vi "Obtain Future.vi"(8 "error in (no error)":errorcluster, 9 "create if not found? (T)":bool=TRUE, 10 "name (unnamed)":string, 11 "Future in":refnum<class "Future.lvclass">) -> (0 "error out":errorcluster, 1 "created new?":bool, 3 "Future out":refnum<class "Future.lvclass">)   [LabVIEW 2017, in "Promise Future.lvlib" / "Future.lvclass"]
uses:
  Future.lvclass
  Future.lvclass/Future.ctl
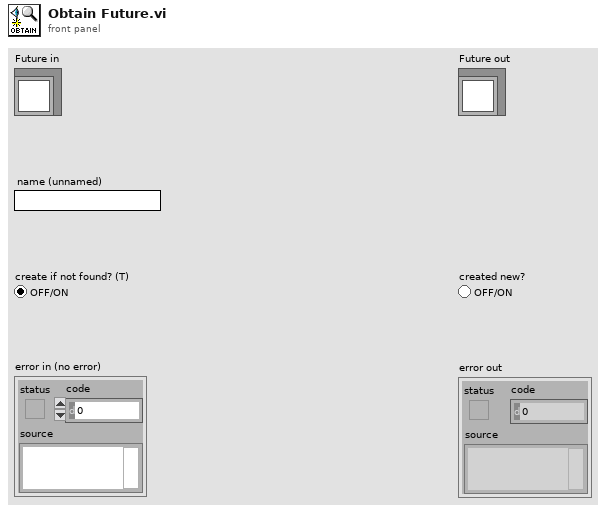
[diagram p1: front panel]
types:
  T1 = cluster{"type specifier VI Refnum (for type only)":refnum<vi>, "Scope":variant}
  T2 = typedef "Semaphore RefNum" = refnum<k1>
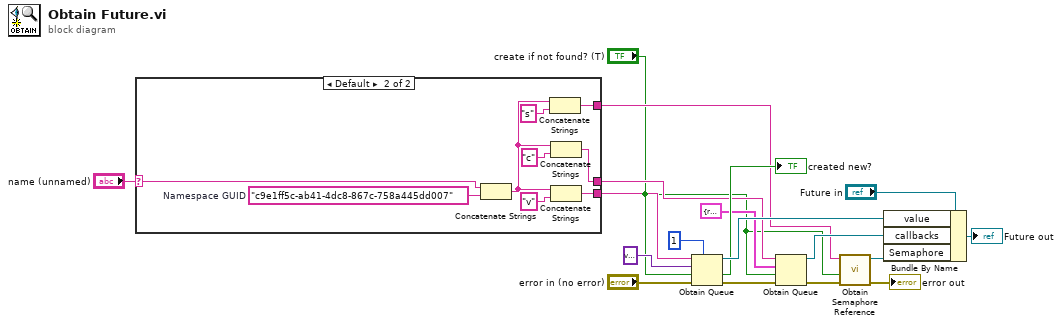
[diagram p0: block diagram]
diagram:
  n1 = case shown="Default" "name (unnamed)" {
    selector: "name (unnamed)" -> [w19 w28]
    tunnel: [w19 w25] -> w7
    tunnel: [w19 w24] -> w6
    tunnel: [w19 w20] -> w2
    frame "" {
    }
    frame Default {
      w27 = "c9e1ff5c-ab41-4dc8-867c-758a445dd007"  # Namespace GUID
      n2 = Concatenate Strings(w28, w27) -> (w22:string)
      n3 = Concatenate Strings(w22, "s" ("string")) -> (w20:string)
      n4 = Concatenate Strings(w22, "c" ("string")) -> (w25:string)
      n5 = Concatenate Strings(w22, "v" ("string")) -> (w24:string)
    }
  }
  n6 = Obtain Queue(max queue size (-1, unlimited)=1, name (unnamed)=w6, element data type=variant, create if not found? (T)="create if not found? (T)", error in (no error)="error in (no error)") -> (queue out=w15:refnum<queue>, created new?=→"created new?":bool, error out=w8:errorcluster)
  n7 = Obtain Queue(name (unnamed)=w7, element data type=T1 {"type specifier VI Refnum (for type only)"=refnum, "Scope"=variant} ("output cluster"), create if not found? (T)="create if not found? (T)", error in (no error)=w8) -> (queue out=w9:refnum<queue>, error out=w4:errorcluster)  [unwired: 1 in, 1 out]
  n8 = call <vilib>:"Obtain Semaphore Reference.vi"("error in (no error)"=w4, "create if not found (T)"="create if not found? (T)", "name (unnamed)"=w2) -> ("error out"=→"error out":errorcluster, "semaphore"=w5:T2)  [unwired: 2 in, 1 out]
  n9 = Bundle By Name(cluster="Future in", "value"=w15, "callbacks"=w9, "Semaphore"=w5) -> (→"Future out":refnum<class "Future.lvclass">)
